vi "SQL_User_Display.vi"() -> (7 "用户信息":string[][](table))   [LabVIEW 2014]
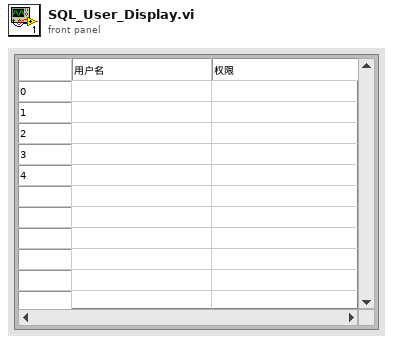
[diagram p1: front panel]
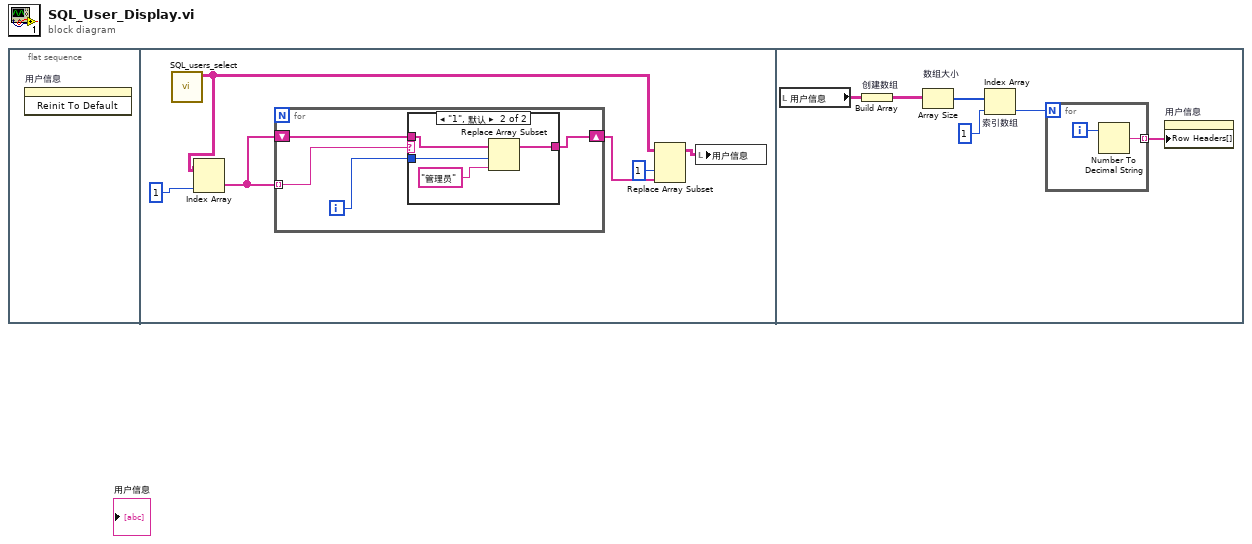
[diagram p0: block diagram]
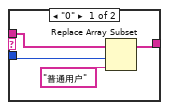
[diagram p2: hidden frame]
diagram:
  n1 = flat-sequence {
    frame #0 {
      n2 = invoke on="用户信息" class="Tbl (严格)" method="Reinit To Default"() -> ()  [unwired: 3 in, 3 out]
    }
    frame #1 {
      n3 = call "SQL_users_select.vi"() -> ("用户信息"=w3:string[][])  [unwired: 10 in, 1 out]
      n4 = Index Array(array=w3, index (col)=1) -> (element=w5:string[])  [unwired: 1 in]
      n5 = for {
        tunnel: w5 -> [w10] mode=indexing
        shift-right: [w7] -> w4
        shift-left: w5 -> [w9]
        i -> [w8]
        n6 = case shown="\"1\", 默认" w10 {
          tunnel: [w11 w18] -> w7
          tunnel: w9 -> [w14 w17]
          tunnel: w8 -> [w13 w16]
          frame "0" {
            n7 = Replace Array Subset(array=w14, new element="普通用户", index=w13) -> (w11:string[])
          }
          frame "1", Default {
            n8 = Replace Array Subset(array=w17, new element="管理员", index=w16) -> (w18:string[])
          }
        }
      }
      n9 = Replace Array Subset(array=w3, new element=w4, index (col)=1 ("禁用的索引 (列)")) -> (w1:string[][])  [unwired: 1 in]
      n10 = local write "用户信息"(w1) -> ()
    }
    frame #2 {
      n11 = local read "用户信息"() -> (w20:string[][])
      n12 = Build Array "创建数组"(w20) -> (w24:string[][][])
      n13 = Array Size "数组大小"(array=w24) -> (size(s)=w23:i32[])
      n14 = Index Array "索引数组"(array=w23, index=1) -> (element=w21:i32)
      n15 = for {
        N: w21 -> [_]
        tunnel: [w25] -> w19 mode=indexing
        i -> [w26]
        n16 = Number To Decimal String(number=w26) -> (decimal integer string=w25:string)  [unwired: 1 in]
      }
      n17 = property on="用户信息" class="Tbl (严格)"("Row Headers[]"=w19) -> ()  [unwired: 2 in, 2 out]
    }
  }
